vi "access_meas_date.vi"() -> (0 "last measurment table":T2(array[cluster]) {"Temperature 2" format="%.2g st. C"}, 1 "last measurment":T1 {"Temperature 2" format="%.2g st. C"})   [LabVIEW 2012]
uses:
  meas_date.vi
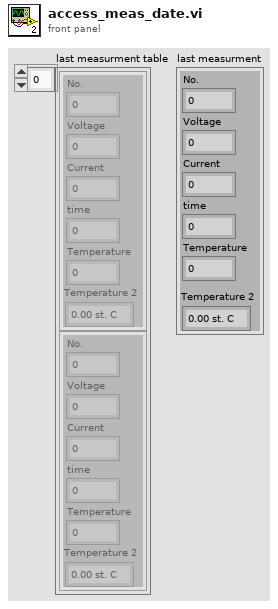
[diagram p1: front panel]
types:
  T1 = cluster{"No.":u64, "Voltage":dbl, "Current":dbl, "time":dbl, "Temperature":dbl, "Temperature 2":dbl}
  T2 = cluster{"No.":u64, "Voltage":dbl, "Current":dbl, "time":dbl, "Temperature":dbl, "Temperature 2":dbl}[]
  T3 = cluster{"VCT measurment's date":cluster{"No.":u64, "Voltage":dbl, "Current":dbl, "time":dbl, "Temperature":dbl, "Temperature 2":dbl}[], "Data":timestamp}[]
  T4 = cluster{"VCT measurment's date":cluster{"No.":u64, "Voltage":dbl, "Current":dbl, "time":dbl, "Temperature":dbl, "Temperature 2":dbl}[], "Data":timestamp}
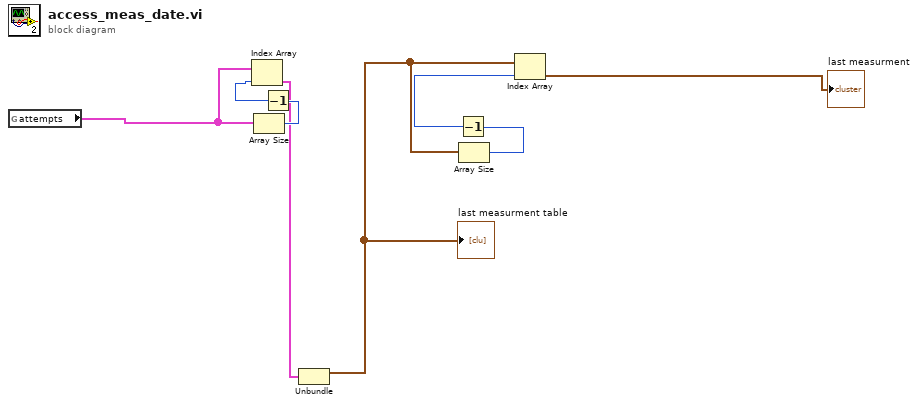
[diagram p0: block diagram]
diagram:
  n1 = global read "meas_date.vi" "attempts"() -> (w8:T3)
  n2 = Array Size(array=w8) -> (size(s)=w7:i32)
  n3 = Decrement(x=w7) -> (x-1=w6:i32)
  n4 = Index Array(array=w8, index=w6) -> (element=w5:T4)
  n5 = Unbundle "Unbundle"(w5) -> ("VCT measurment's date"=w1:T2)  [unwired: 1 out]
  "last measurment table" <- w1
  n6 = Array Size(array=w1) -> (size(s)=w4:i32)
  n7 = Decrement(x=w4) -> (x-1=w3:i32)
  n8 = Index Array(array=w1, index=w3) -> (element=→"last measurment":T1)
